vi "Main-Markov Estimation.vi"() -> ()   [LabVIEW 2014]
panel:
  in  "parameter":T1
  in  "Tab":enum32{"Interference", "Delay"}(tab)
  in  "device names":refnum<k15>="192.168.10.2"
  in  "Wifi Channel":i32=3
  out "USRP error":errorcluster
  out "coerced carrier frequency":dbl=2421999999.997206 format="%#_6p"
  in  "SamplingTimes":i32=100
  in  "Sampling Para.":T1={"Method"=enum."Binary", "offset"=0, "threshold"=1.0, "step"=1.0}
  in  "Number of Samplings":i32=100
  in  "UDP parameter":T2={"remote IP Address"="192.168.1.101", "remote port"=54322, "local port(Tx)"=54321, "local port(Rx)"=54323}
  out "UDP error":errorcluster
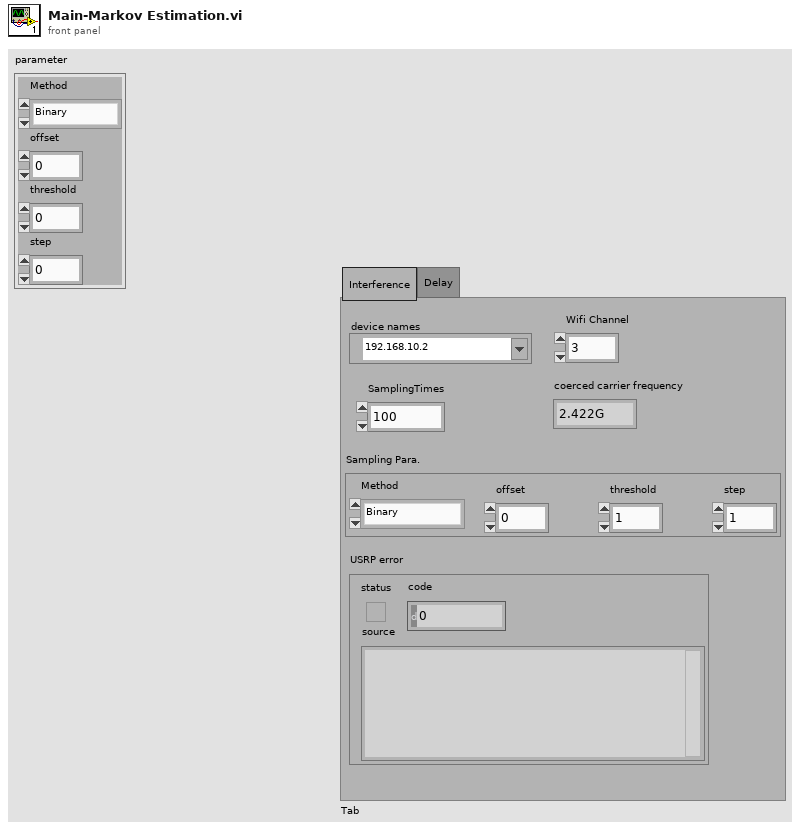
[diagram p1: front panel]
types:
  T1 = cluster{"Method":enum16{"Binary", "Uniform"}, "offset":i32, "threshold":dbl, "step":dbl}
  T2 = cluster{"remote IP Address":string, "remote port":u16, "local port(Tx)":u16, "local port(Rx)":u16}
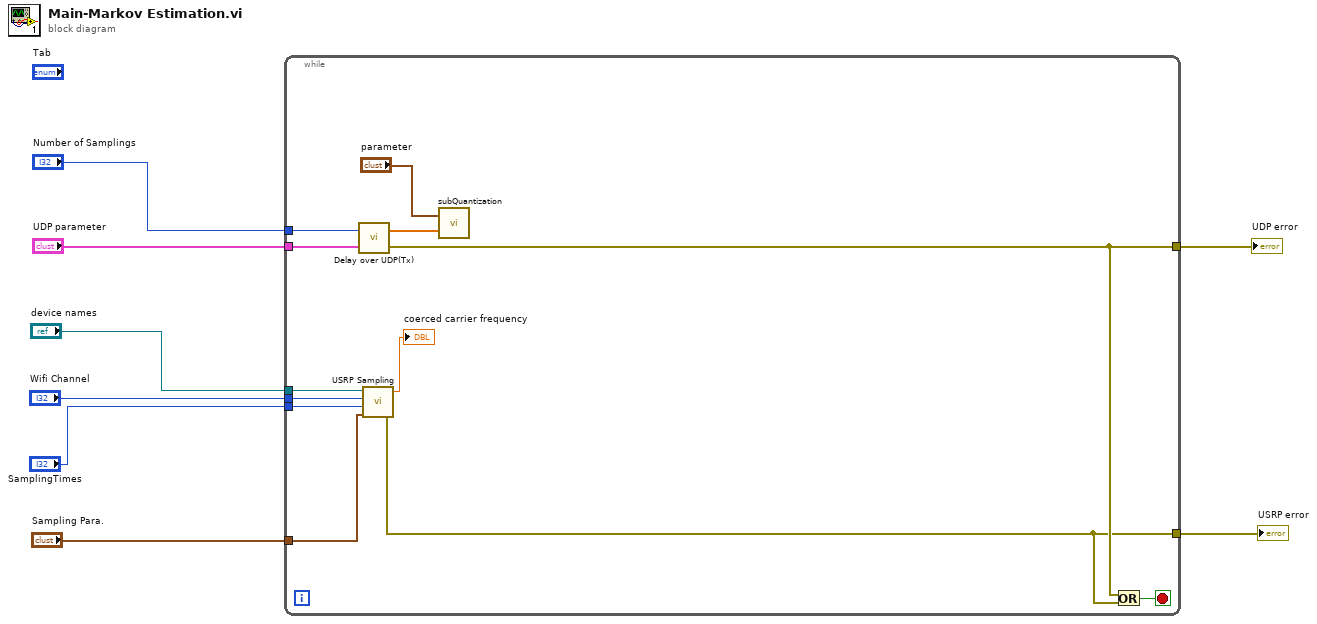
[diagram p0: block diagram]
diagram:
  n1 = while {
    tunnel: "Number of Samplings" -> [w20]
    tunnel: "UDP parameter" -> [w19]
    tunnel: "device names" -> [w18]
    tunnel: "Wifi Channel" -> [w17]
    tunnel: "SamplingTimes" -> [w16]
    tunnel: "Sampling Para." -> [w15]
    tunnel: [w10] -> w2
    tunnel: [w9] -> w1
    stop <- w11 stop-if-true
    n2 = call "Delay over UDP(Tx).vi"("parameter"=w19, "Number of Samplings"=w20) -> ("error out"=w10:errorcluster, "Output"=w12:dbl[])
    n3 = call "USRP Sampling.vi"("parameter"=w15, "SamplingTimes"=w16, "Wifi Channel"=w17, "device names"=w18) -> ("error out"=w9:errorcluster, "coerced carrier frequency"=→"coerced carrier frequency":dbl)  [unwired: 1 out]
    n4 = call "subQuantization.vi"("input"=w12, "parameter"="parameter") -> ()  [unwired: 2 out]
    n5 = Or(x=w10, y=w9) -> (x .or. y?=w11:bool)
  }
  "UDP error" <- w2
  "USRP error" <- w1
